vi "FINAL_IMAGE CHECKING.vi"() -> ()   [LabVIEW 2018]
uses:
  <vilib>/vision/Pattern Matching.llb/IMAQ GM Match Report.ctl
  <vilib>/userdefined/High Color/IMAQdx.ctl
  Underlying VI's/Webcam FGV Low level ver/State control.ctl
panel:
  out "Calibrated Matches (Pattern Matching 1)":T1[](array[typedef]) {"Correlation Score" format="%.2f"; "Target Template Curve Score" format="%.2f"; "Template Target Curve Score" format="%.2f"; "Bounding Box"."y" format="%.2f"; "Bounding Box"."x" format="%.2f"; "Position"."y" format="%.2f"; "Position"."x" format="%.2f"; "Score" format="%.2f"; "Scale" format="%.2f"; "Angle" format="%.2f"; "Occlusion %" format="%.2f"}
  out "Obj coordinates":cluster{"x":sgl, "y":sgl, "x":sgl, "y":sgl}
  out "error out":errorcluster
  out "Image":T2(plugin-control)
  out "Shape Report (calibrated)":T3(array[cluster])
  in  "Mode":enum16{"Ball", "Soap", "Gel", "Pipe", "None"}(ring)
  out "Number of Matches (Color Pattern Matching 1)":i32
  in  "Stop (F)":bool
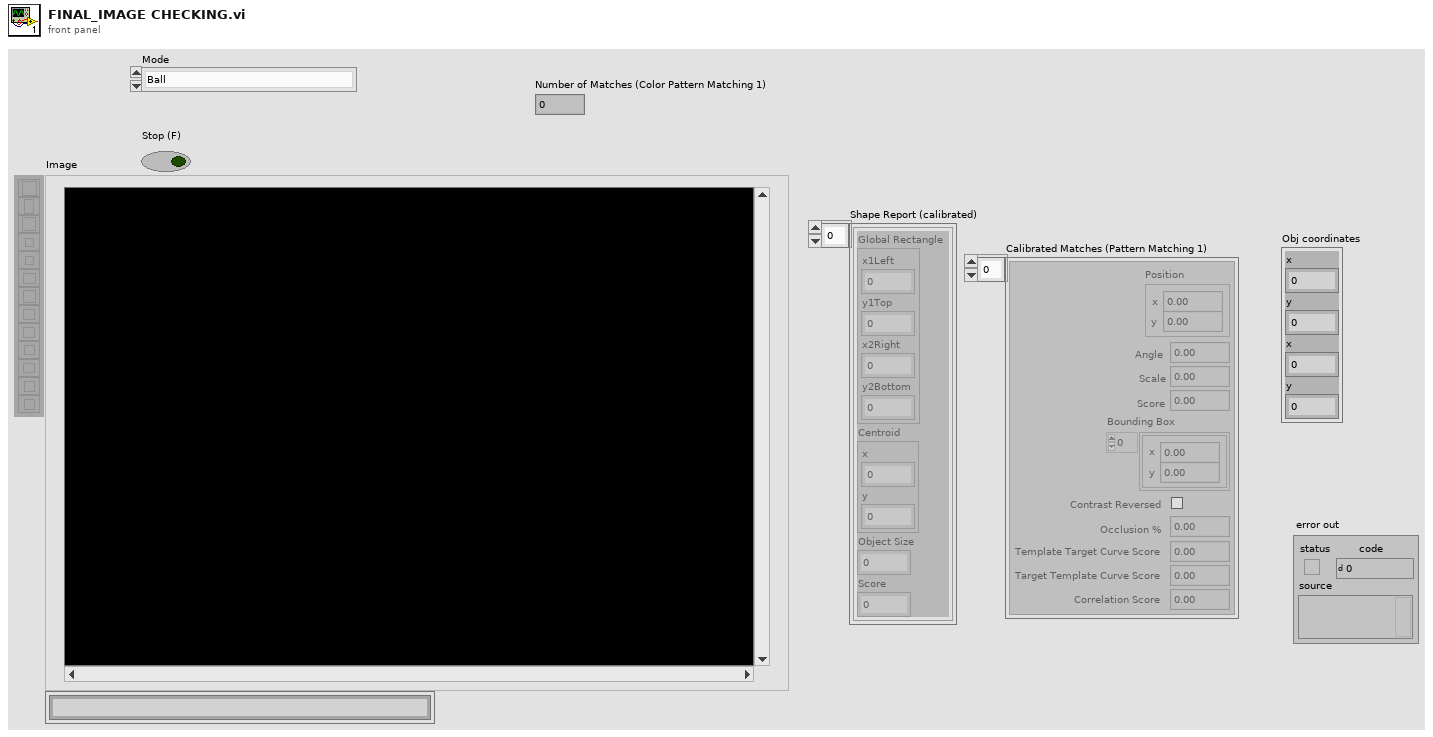
[diagram p1: front panel]
types:
  T1 = typedef "IMAQ GM Match Report.ctl" = cluster{"Position":cluster{"x":sgl, "y":sgl}, "Angle":sgl, "Scale":sgl, "Score":sgl, "Bounding Box":cluster{"x":sgl, "y":sgl}[], "Contrast Reversed":bool, "Occlusion %":sgl, "Template Target Curve Score":sgl, "Target Template Curve Score":sgl, "Correlation Score":sgl}
  T2 = typedef "IMAQ Image.ctl" = refnum<image>
  T3 = cluster{"Global Rectangle":cluster{"x1Left":i32, "y1Top":i32, "x2Right":i32, "y2Bottom":i32}, "Centroid":cluster{"x":sgl, "y":sgl}, "Object Size":u32, "Score":dbl}[]
  T4 = typedef "State control.ctl" = enum16{"Initialise", "Start camera", "Continuous Acquisition ", "Stop camera", "Dispose all"}
  T5 = typedef "IMAQdx.ctl" = refnum<k21>
  T6 = cluster{"Calibrated Matches (Pattern Matching 1)[0]":T1, "Calibrated Matches (Pattern Matching 1)[1]":T1, "Calibrated Matches (Pattern Matching 1)[2]":T1, "Calibrated Matches (Pattern Matching 1)[3]":T1, "Calibrated Matches (Pattern Matching 1)[4]":T1, "Calibrated Matches (Pattern Matching 1)[5]":T1, "Calibrated Matches (Pattern Matching 1)[6]":T1, "Calibrated Matches (Pattern Matching 1)[7]":T1, "Calibrated Matches (Pattern Matching 1)[8]":T1}
  T7 = cluster{"Shape Report (calibrated) (Shape Matching 1)[0]":cluster{"Global Rectangle":cluster{"x1Left":i32, "y1Top":i32, "x2Right":i32, "y2Bottom":i32}, "Centroid":cluster{"x":sgl, "y":sgl}, "Object Size":u32, "Score":dbl}, "Shape Report (calibrated) (Shape Matching 1)[1]":cluster{"Global Rectangle":cluster{"x1Left":i32, "y1Top":i32, "x2Right":i32, "y2Bottom":i32}, "Centroid":cluster{"x":sgl, "y":sgl}, "Object Size":u32, "Score":dbl}, "Shape Report (calibrated) (Shape Matching 1)[2]":cluster{"Global Rectangle":cluster{"x1Left":i32, "y1Top":i32, "x2Right":i32, "y2Bottom":i32}, "Centroid":cluster{"x":sgl, "y":sgl}, "Object Size":u32, "Score":dbl}, "Shape Report (calibrated) (Shape Matching 1)[3]":cluster{"Global Rectangle":cluster{"x1Left":i32, "y1Top":i32, "x2Right":i32, "y2Bottom":i32}, "Centroid":cluster{"x":sgl, "y":sgl}, "Object Size":u32, "Score":dbl}, "Shape Report (calibrated) (Shape Matching 1)[4]":cluster{"Global Rectangle":cluster{"x1Left":i32, "y1Top":i32, "x2Right":i32, "y2Bottom":i32}, "Centroid":cluster{"x":sgl, "y":sgl}, "Object Size":u32, "Score":dbl}, "Shape Report (calibrated) (Shape Matching 1)[5]":cluster{"Global Rectangle":cluster{"x1Left":i32, "y1Top":i32, "x2Right":i32, "y2Bottom":i32}, "Centroid":cluster{"x":sgl, "y":sgl}, "Object Size":u32, "Score":dbl}, "Shape Report (calibrated) (Shape Matching 1)[6]":cluster{"Global Rectangle":cluster{"x1Left":i32, "y1Top":i32, "x2Right":i32, "y2Bottom":i32}, "Centroid":cluster{"x":sgl, "y":sgl}, "Object Size":u32, "Score":dbl}, "Shape Report (calibrated) (Shape Matching 1)[7]":cluster{"Global Rectangle":cluster{"x1Left":i32, "y1Top":i32, "x2Right":i32, "y2Bottom":i32}, "Centroid":cluster{"x":sgl, "y":sgl}, "Object Size":u32, "Score":dbl}, "Shape Report (calibrated) (Shape Matching 1)[8]":cluster{"Global Rectangle":cluster{"x1Left":i32, "y1Top":i32, "x2Right":i32, "y2Bottom":i32}, "Centroid":cluster{"x":sgl, "y":sgl}, "Object Size":u32, "Score":dbl}}
  T8 = cluster{"Global Rectangle":cluster{"x1Left":i32, "y1Top":i32, "x2Right":i32, "y2Bottom":i32}, "Centroid":cluster{"x":sgl, "y":sgl}, "Object Size":u32, "Score":dbl}
  T9 = cluster{"x1Left":i32, "y1Top":i32, "x2Right":i32, "y2Bottom":i32}
  T10 = cluster{"x1Left":sgl, "y1Top":sgl, "x2Right":sgl, "y2Bottom":sgl}
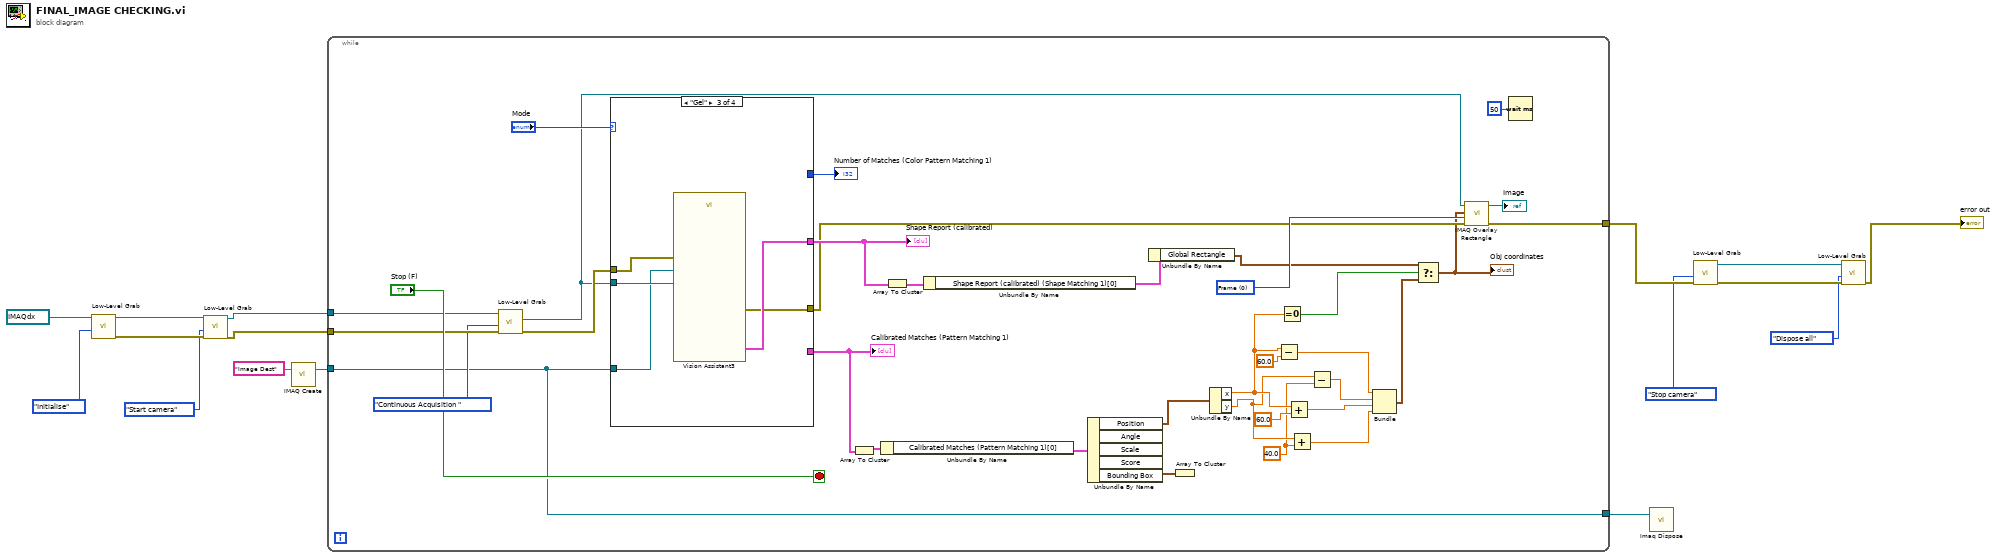
[diagram p0: block diagram]
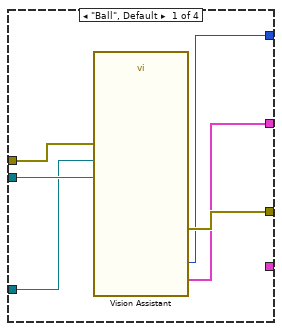
[diagram p2: hidden frame]
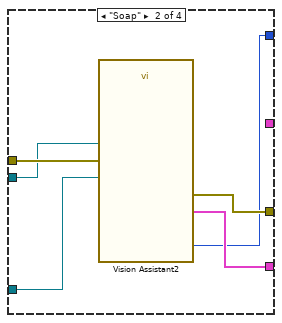
[diagram p3: hidden frame]
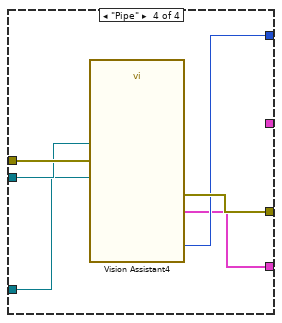
[diagram p4: hidden frame]
diagram:
  n1 = call "Low-Level Grab.vi"("States"=State_control."Initialise", "Session In"=T5 "cam0") -> ("error out"=w14:errorcluster, "Session Out"=w15:T5)  [unwired: 7 in, 1 out]
  n2 = call "Low-Level Grab.vi"("error in (no error)"=w14, "States"=State_control."Start camera", "Session In"=w15) -> ("error out"=w11:errorcluster, "Session Out"=w4:T5)  [unwired: 6 in, 1 out]
  n3 = call "IMAQ Create"("Image Name"="Image Dest") -> ("New Image"=w2:T2)  [unwired: 4 in, 1 out]
  n4 = while {
    tunnel: w11 -> [w40]
    tunnel: [w37] -> w8
    tunnel: w4 -> [w35]
    tunnel: w2 -> [w34]
    tunnel: [w34] -> w1
    stop <- "Stop (F)" stop-if-true
    w19 = sgl 40.0 ("y")
    w45 = u32 0 items=["Frame", "Fill", "Highlight"] ("Drawing Mode (Frame)")
    n5 = call "Low-Level Grab.vi"("error in (no error)"=w40, "States"=State_control."Continuous Acquisition ", "Session In"=w35) -> ("error out"=w38:errorcluster, "Image Out"=w36:T2)  [unwired: 6 in, 1 out]
    n6 = case shown="\"Gel\"" "Mode" {
      tunnel: [w55 _ w68 _] -> w48
      tunnel: w38 -> [w57 w63 w67 w74]
      tunnel: [w56 w62 w66 w73] -> w44
      tunnel: w36 -> [w54 w61 w65 w72]
      tunnel: w34 -> [w53 w60 w64 w71]
      tunnel: [w52 w58 _ w70] -> w33
      tunnel: [_ w59 _ w69] -> w32
      frame "Ball", Default {
        n7 = call "Vision Assistant"("Image In"=w54, "Image Dst"=w53, "error in"=w57) -> ("Number of Matches (Shape Matching 1)"=w52:i32, "Shape Report (calibrated) (Shape Matching 1)"=w55:T3, "error out"=w56:errorcluster)  [unwired: 21 in, 1 out]
      }
      frame "Soap" {
        n8 = call "Vision Assistant2"("Image In"=w61, "Image Dst"=w60, "error in"=w63) -> ("Number of Matches (Pattern Matching 1)"=w58:i32, "Calibrated Matches (Pattern Matching 1)"=w59:T1[], "error out"=w62:errorcluster)  [unwired: 21 in, 1 out]
      }
      frame "Gel" {
        n9 = call "Vision Assistant3"("Image In"=w65, "Image Dst"=w64, "error in"=w67) -> ("Shape Report (calibrated) (Shape Matching 1)"=w68:T3, "error out"=w66:errorcluster)  [unwired: 21 in, 2 out]
      }
      frame "Pipe" {
        n10 = call "Vision Assistant4"("Image In"=w72, "Image Dst"=w71, "error in"=w74) -> ("Number of Matches (Pattern Matching 1)"=w70:i32, "Calibrated Matches (Pattern Matching 1)"=w69:T1[], "error out"=w73:errorcluster)  [unwired: 21 in, 1 out]
      }
    }
    "Number of Matches (Color Pattern Matching 1)" <- w33
    "Shape Report (calibrated)" <- w48
    "Calibrated Matches (Pattern Matching 1)" <- w32
    n11 = Array To Cluster(array=w32) -> (cluster=w31:T6)
    n12 = Unbundle By Name(w31) -> ("Calibrated Matches (Pattern Matching 1)[0]"=w30:T1)
    n13 = Array To Cluster(array=w48) -> (cluster=w47:T7)
    n14 = Unbundle By Name(w47) -> ("Shape Report (calibrated) (Shape Matching 1)[0]"=w18:T8)
    n15 = Unbundle By Name(w30) -> ("Position"=w28:cluster{"x":sgl, "y":sgl}, "Bounding Box"=w29:cluster{"x":sgl, "y":sgl}[])  [unwired: 3 out]
    n16 = Unbundle By Name(w18) -> ("Global Rectangle"=w17:T9)
    n17 = Array To Cluster(array=w29) -> ()  [unwired: 1 out]
    n18 = Unbundle By Name(w28) -> ("x"=w23:sgl, "y"=w21:sgl)
    n19 = Subtract(x=w23, y=sgl 60.0) -> (x-y=w22:sgl)
    n20 = Equal To 0?(x=w23) -> (x = 0?=w42:bool)
    n21 = Add(x=w23, y=sgl 60.0) -> (x+y=w26:sgl)
    n22 = Add(x=w21, y=w19) -> (x+y=w25:sgl)
    n23 = Subtract(x=w21, y=w19) -> (x-y=w20:sgl)
    n24 = Bundle(w22, w20, w26, w25) -> (w41:cluster{sgl, sgl, sgl, sgl})  [unwired: 1 in]
    n25 = Select(t=w17, s=w42, f=w41) -> (s? t:f=w43:T10)
    "Obj coordinates" <- w43
    n26 = call "IMAQ Overlay Rectangle"("error in (no error)"=w44, "Drawing Mode (Frame)"=w45, "Rectangle"=w43, "Image"=w36) -> ("error out"=w37:errorcluster, "Image Out"=→"Image":T2)  [unwired: 6 in]
    n27 = Wait (ms)(milliseconds to wait=u32 50) -> ()  [unwired: 1 out]
  }
  n28 = call "Imaq Dispose"("Image"=w1) -> ()  [unwired: 5 in, 1 out]
  n29 = call "Low-Level Grab.vi"("error in (no error)"=w8, "States"=State_control."Stop camera") -> ("error out"=w9:errorcluster, "Session Out"=w10:T5)  [unwired: 7 in, 1 out]
  n30 = call "Low-Level Grab.vi"("error in (no error)"=w9, "States"=State_control."Dispose all", "Session In"=w10) -> ("error out"=→"error out":errorcluster)  [unwired: 6 in, 2 out]
